vi "InitGlobals.vi"(8 "Error In":errorcluster) -> (0 "Error Out":errorcluster)   [LabVIEW 2017, in "Client.lvlib" / "CommsFrameWork.lvlib"]
uses:
  CommsFrameWork.lvlib
  ClientGlobals.vi
  Client.lvlib
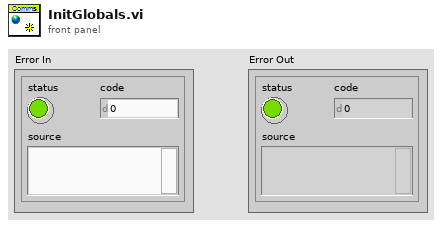
[diagram p1: front panel]
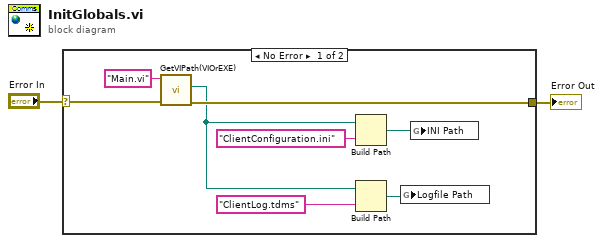
[diagram p0: block diagram]
diagram:
  n1 = case shown="No Error" "Error In" {
    selector: "Error In" -> [w10 w11]
    tunnel: [w7 w11] -> w1
    frame No Error {
      n2 = call "GetVIPath(VIOrEXE).vi"("error in (no error)"=w10, "VI Name to Find"="Main.vi") -> ("error out"=w7:errorcluster, "VI or executable installation directory"=w3:path)  [unwired: 7 in, 1 out]
      n3 = Build Path(base path=w3, name or relative path="ClientConfiguration.ini") -> (appended path=w9:path)
      n4 = Build Path(base path=w3, name or relative path="ClientLog.tdms") -> (appended path=w4:path)
      n5 = global write "ClientGlobals.vi" "Logfile Path"(w4) -> ()
      n6 = global write "ClientGlobals.vi" "INI Path"(w9) -> ()
    }
    frame Error {
    }
  }
  "Error Out" <- w1
